vi "Set Out.vi"(8 "error in (no error)":errorcluster, 10 "Output value":refnum<class "Output Value.lvclass">, 11 "IPS120 in":refnum<class "IPS120.lvclass">) -> (0 "error out":errorcluster, 3 "IPS120 out":refnum<class "IPS120.lvclass">)   [LabVIEW 2018, in "IPS120.lvclass"]
uses:
  IPS120.lvclass
  C:/github/NHMFL_Core/Libraries/Instruments/VISA Instrument/VISA Instrument.lvclass
  Utilities/Output Value/Output Value.lvclass
  Results/Set Sweep/Set Sweep.lvclass
  VISA Instrument/VISA Instrument.lvclass/VISA Instrument.ctl
  VISA Instrument/Read VISA resource.vi
  VISA Instrument/Write VISA resource.vi
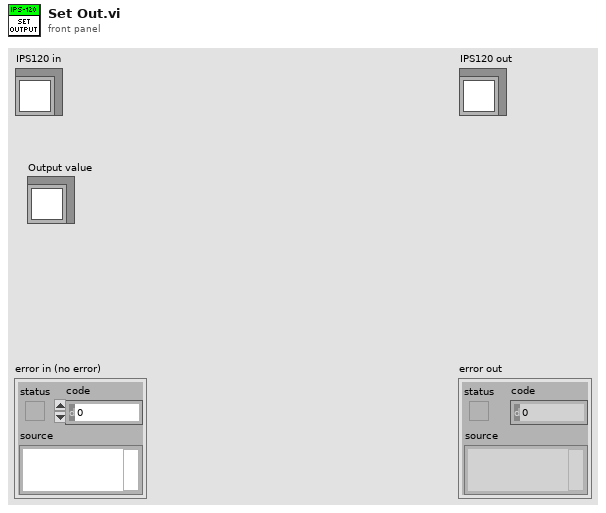
[diagram p1: front panel]
types:
  T1 = typedef "Set Output.ctl" = cluster{"Set point":dbl, "Sweep rate":dbl, "Sweep action":T2}
  T2 = typedef "Sweep Action.ctl" = enum16{"To set point", "To zero", "Hold", "Clamp"}
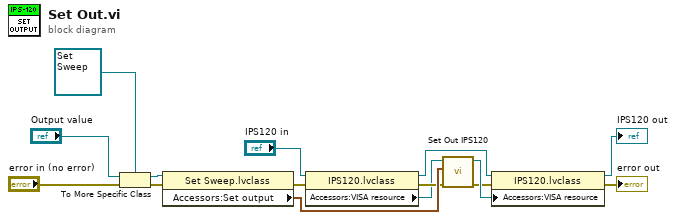
[diagram p0: block diagram]
diagram:
  n1 = To More Specific Class(target class=refnum<class "Set Sweep.lvclass"> refnum ("Set Sweep.lvclass"), reference="Output value", error in="error in (no error)") -> (specific class reference=w9:refnum<class "Set Sweep.lvclass">, error out=w6:errorcluster)
  n2 = property class="Set Sweep.lvclass"(reference=w9, error in=w6) -> (error out=w14:errorcluster, "Accessors:Set output"=w5:T1)  [unwired: 1 out]
  n3 = property class="IPS120.lvclass"(reference="IPS120 in", error in=w14) -> (reference out=w15:refnum<class "IPS120.lvclass">, error out=w4:errorcluster, "Accessors:VISA resource"=w3:refnum<visa-resource-name>)
  n4 = call "Set Out IPS120.vi"("Error In"=w4, "Set output"=w5, "VISA resource name"=w3) -> ("Error Out"=w1:errorcluster, "VISA resource name out"=w2:refnum<visa-resource-name>)  [unwired: 7 in]
  n5 = property class="IPS120.lvclass"(reference=w15, error in=w1, "Accessors:VISA resource"=w2) -> (reference out=→"IPS120 out":refnum<class "IPS120.lvclass">, error out=→"error out":errorcluster)
